vi "N_forsed_bits.vi"(3 "IN":u32 format="%b") -> (1 "N_forsed_bits":u32)   [LabVIEW 2019, in "Logik.lvlib"]
uses:
  Logik.lvlib
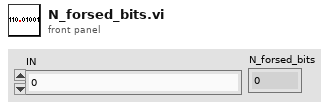
[diagram p1: front panel]
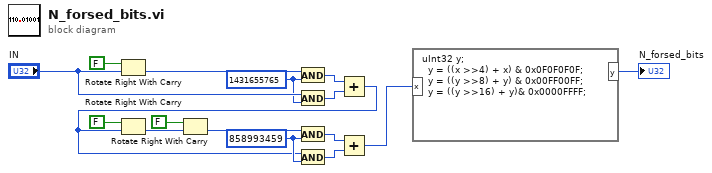
[diagram p0: block diagram]
diagram:
  w8 = u32 858993459 ("y")
  w12 = u32 1431655765 ("y")
  n1 = Rotate Right With Carry(2:"IN", 3:FALSE ("carry")) -> (0:w14:u32)  [unwired: 1 out]
  n2 = And(x=w14, y=w12) -> (x .and. y?=w11:u32)
  n3 = And(x="IN", y=w12) -> (x .and. y?=w10:u32)
  n4 = Add(x=w11, y=w10) -> (x+y=w5:u32)
  n5 = Rotate Right With Carry(2:w5, 3:FALSE ("carry")) -> (0:w2:u32)  [unwired: 1 out]
  n6 = Rotate Right With Carry(2:w2, 3:FALSE ("carry")) -> (0:w4:u32)  [unwired: 1 out]
  n7 = And(x=w4, y=w8) -> (x .and. y?=w7:u32)
  n8 = And(x=w5, y=w8) -> (x .and. y?=w6:u32)
  n9 = Add(x=w7, y=w6) -> (x+y=w1:u32)
  n10 = formula code="uInt32 y;\n  y = ((x >>4) + x) & 0x0F0F0F0F;\n  y = ((y >>8) + y) & 0x00FF00FF;\n  y = ((y >>16) + y)& 0x0000FFFF;"("x"=w1) -> ("y"=→"N_forsed_bits":u32)
